vi "Simulation Interface.vi"(8 "error in (no error)":errorcluster) -> (0 "error out":errorcluster)   [LabVIEW 2017]
doc: "A main program that is run to test ATM algorithms in a software-only environment."
uses:
  View Model/Controls/Interface.ctl
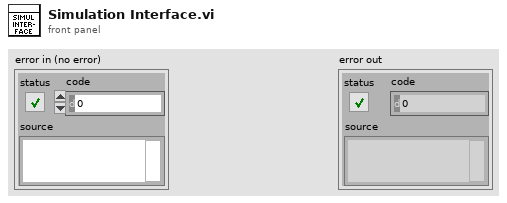
[diagram p1: front panel]
types:
  T1 = typedef "View Model.ctl" = cluster{"Shared Model":T2, "Error Model":T3, "Config Model":T4, "Controller Model":T5}
  T2 = typedef "Shared Model.ctl" = cluster{"Stop":refnum<user-event>, "Stop DVR":refnum<data-value>}
  T3 = typedef "Error Model.ctl" = cluster{"Error":refnum<user-event>}
  T4 = typedef "Config Model.ctl" = cluster{"Config CMD":refnum<user-event>}
  T5 = typedef "Controller Model.ctl" = cluster{"Deposit Received":refnum<user-event>, "Funds Dispensed":refnum<user-event>, "Overhead DVR":refnum<data-value>, "Entered Num":refnum<user-event>, "Card Read":refnum<user-event>, "Transaction":refnum<user-event>}
  T6 = typedef "Interface.ctl" = enum16{"Simulated", "Hardware"}
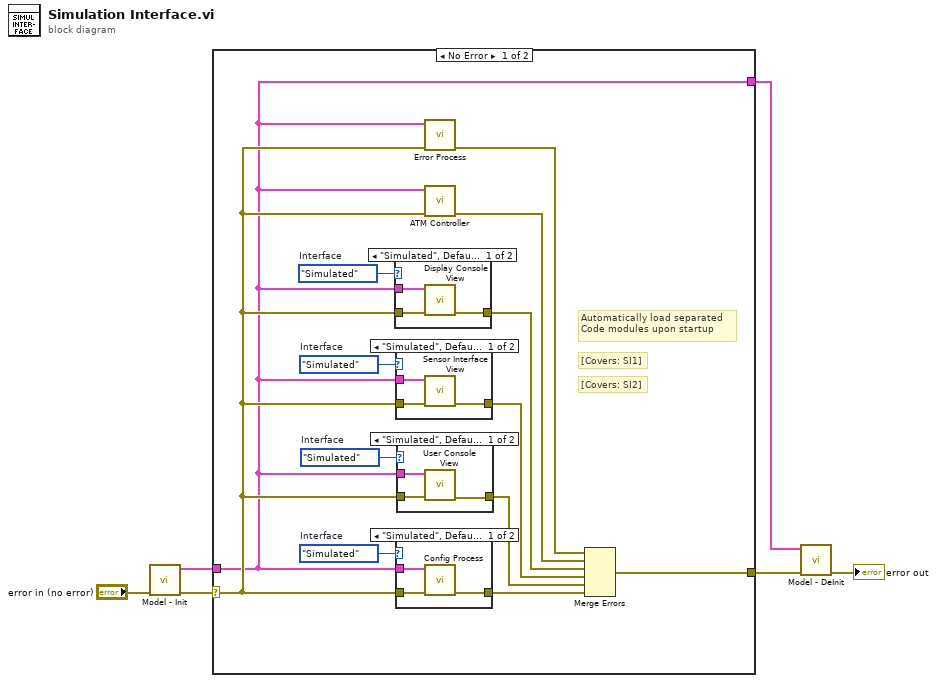
[diagram p0: block diagram]
diagram:
  n1 = call "Model - Init.vi"("error in (no error)"="error in (no error)") -> ("error out"=w6:errorcluster, "View Model"=w4:T1)  [unwired: 9 in]
  n2 = case shown="No Error" w6 {
    selector: w6 -> [w15 w36]
    tunnel: w4 -> [w7 w37]
    tunnel: [w8 w36] -> w3
    tunnel: [w7 w37] -> w1
    frame No Error {
      w16 = Interface."Simulated"  # Interface
      w17 = Interface."Simulated"  # Interface
      w18 = Interface."Simulated"  # Interface
      w19 = Interface."Simulated"  # Interface
      # "Automatically load separated\nCode modules upon startup"
      # "[Covers: SI2]"
      # "[Covers: SI1]"
      n3 = case shown="\"Simulated\", Default" w16 {
        tunnel: w15 -> [w22 w23]
        tunnel: [w21 w23] -> w11
        tunnel: w7 -> [w20 _]
        frame "Simulated", Default {
          n4 = call "Display Console View.vi"("error in (no error)"=w22, "View Model"=w20) -> ("error out"=w21:errorcluster)  [unwired: 9 in]
        }
        frame "Hardware" {
        }
      }
      n5 = case shown="\"Simulated\", Default" w17 {
        tunnel: w15 -> [w26 w27]
        tunnel: [w25 w27] -> w12
        tunnel: w7 -> [w24 _]
        frame "Simulated", Default {
          n6 = call "Sensor Interface View.vi"("error in (no error)"=w26, "View Model"=w24) -> ("error out"=w25:errorcluster)  [unwired: 9 in]
        }
        frame "Hardware" {
        }
      }
      n7 = case shown="\"Simulated\", Default" w19 {
        tunnel: w15 -> [w34 w35]
        tunnel: w7 -> [w33 _]
        tunnel: [w32 w35] -> w14
        frame "Simulated", Default {
          n8 = call "Config Process.vi"("error in (no error)"=w34, "View Model"=w33) -> ("error out"=w32:errorcluster)  [unwired: 9 in]
        }
        frame "Hardware" {
        }
      }
      n9 = case shown="\"Simulated\", Default" w18 {
        tunnel: w15 -> [w30 w31]
        tunnel: [w29 w31] -> w13
        tunnel: w7 -> [w28 _]
        frame "Simulated", Default {
          n10 = call "User Console View.vi"("error in (no error)"=w30, "View Model"=w28) -> ("error out"=w29:errorcluster)  [unwired: 9 in]
        }
        frame "Hardware" {
        }
      }
      n11 = call "Error Process.vi"("error in (no error)"=w15, "View Model"=w7) -> ("error out"=w9:errorcluster)  [unwired: 9 in]
      n12 = call "ATM Controller.vi"("error in (no error)"=w15, "View Model"=w7) -> ("error out"=w10:errorcluster)  [unwired: 9 in]
      n13 = Merge Errors(w9, w10, w11, w12, w13, w14) -> (w8:errorcluster)
    }
    frame Error {
    }
  }
  n14 = call "Model - DeInit.vi"("error in (no error)"=w3, "View Model"=w1) -> ("error out"=→"error out":errorcluster)  [unwired: 9 in]
